vi "Get Routing Channel by Name.vi"(8 "error in":errorcluster, 10 "channel name":string, 11 "routing channels in":T1 format="%.0x") -> (0 "error out":errorcluster, 2 "routing channel":T1 format="%.0x", 3 "routing channels out":T1 format="%.0x")   [LabVIEW 2020, in "Routing and Faulting Scripting.lvlib"]
doc: "Returns the routing channel with a specified name."
uses:
  Routing and Faulting Scripting.lvlib
  <vilib>/NI VeriStand/Custom Device API/Custom Device Item Ref.ctl
  <vilib>/NI VeriStand/Custom Device API/Custom Device API.lvlib
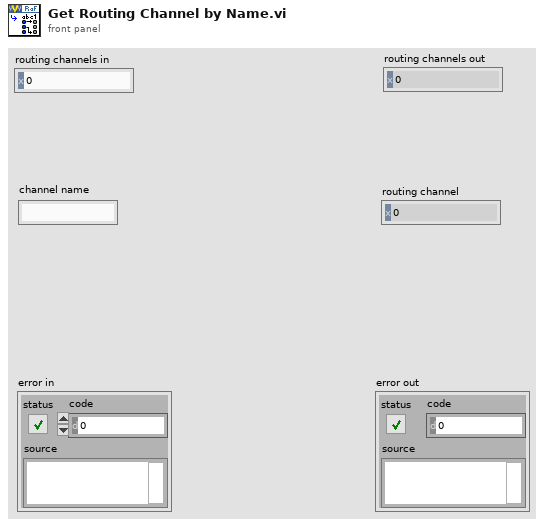
[diagram p1: front panel]
types:
  T1 = typedef "Custom Device API.lvlib/Custom Device Item Ref.ctl" = u64
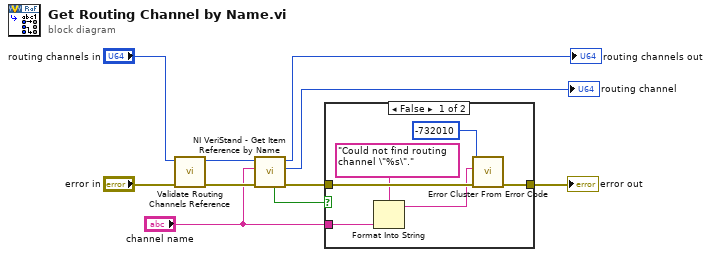
[diagram p0: block diagram]
diagram:
  n1 = call "Validate Routing Channels Reference.vi"("error in"="error in", "routing channels in"="routing channels in") -> ("error out"=w7:errorcluster, "routing channels out"=w5:T1)  [unwired: 8 in]
  n2 = call <vilib>:"NI VeriStand - Get Item Reference by Name.vi"("error in (no error)"=w7, "Item Name"="channel name", "Parent Ref in"=w5) -> ("error out"=w3:errorcluster, "Item Ref"=→"routing channel":T1, "Parent Ref out"=→"routing channels out":T1, "Found"=w4:bool)  [unwired: 5 in]
  n3 = case shown="False" w4 {
    tunnel: w3 -> [w14 w17]
    tunnel: [w16 w17] -> w2
    tunnel: "channel name" -> [w13 _]
    frame False {
      n4 = Format Into String(format string="Could not find routing channel \"%s\".", w13) -> (resulting string=w12:string)  [unwired: 2 in, 1 out]
      n5 = call <vilib>:"Error Cluster From Error Code.vi"("error in (no error)"=w14, "error message (\"\")"=w12, "error code (0)"=-732010) -> ("error out"=w16:errorcluster)  [unwired: 6 in]
    }
    frame True {
    }
  }
  "error out" <- w2
